vi "test Close References.vi"(8 "error in":errorcluster) -> (0 "error out":errorcluster)   [LabVIEW 2020, in "ase.test.lvlib"]
uses:
  ase.test.lvlib
  <vilib>/addons/_JKI Toolkits/Caraya/classes/Test/Test.lvclass
  <vilib>/addons/_JKI Toolkits/Caraya/classes/Assert/Assert.lvclass
  ase/ase/ase.lvclass
  ase/ase/Standard Output.ctl
  ase/ase/Standard Error.ctl
  ase/ase/Did Exit.ctl
  ase/ase/Event References.ctl
  <vilib>/addons/_JKI Toolkits/Caraya/classes/Assert/Assert Not Error.vi
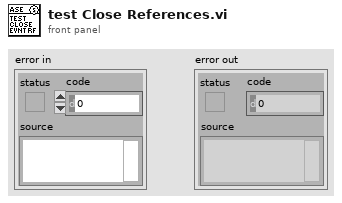
[diagram p1: front panel]
types:
  T1 = typedef "ase.lvlib/ase.lvclass/Event References.ctl" = cluster{"Standard Output":refnum<user-event>, "Standard Error":refnum<user-event>, "Did Exit":refnum<user-event>}
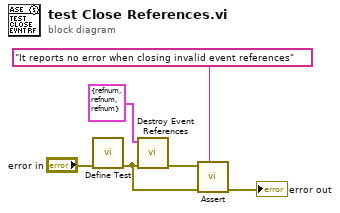
[diagram p0: block diagram]
diagram:
  n1 = call <vilib>:"Define Test.vi"("error in (no error)"="error in") -> ("error out"=w1:errorcluster)  [unwired: 9 in, 1 out]
  n2 = call "Destroy Event References.vi"("error in"=w1, "Event References"=T1 {"Standard Output"=refnum, "Standard Error"=refnum, "Did Exit"=refnum}) -> ("error out"=w2:errorcluster)  [unwired: 9 in]
  n3 = call-poly <vilib>:"Assert.vi"("Label"="It reports no error when closing invalid event references", "error in (no error)"=w1, "Not Error?"=w2) -> ("error out"=→"error out":errorcluster)  [unwired: 7 in, 1 out]
